vi "Add Frame.vi"(7 "Highlight? (F)":bool, 8 "error in":errorcluster, 10 "Name":string, 11 "Port Ref":T1 format="%.0x") -> (0 "error out":errorcluster, 2 "Newly Created?":bool, 3 "Frame Ref out":T1 format="%.0x")   [LabVIEW 2020, in "Ballard ARINC 429 Scripting.lvlib"]
uses:
  Ballard ARINC 429 Scripting.lvlib
  <vilib>/NI VeriStand/Custom Device API/Custom Device Item Ref.ctl
  Constants.vi
  <vilib>/NI VeriStand/Custom Device API/Custom Device API.lvlib
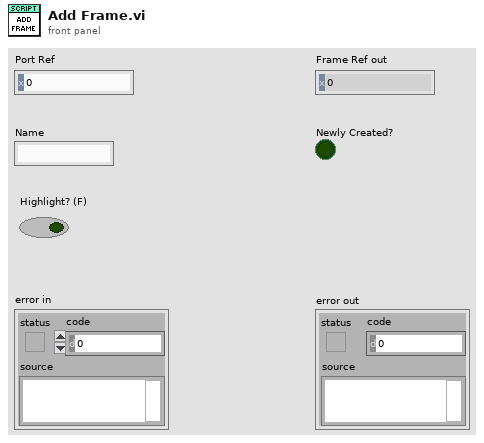
[diagram p1: front panel]
types:
  T1 = typedef "Custom Device API.lvlib/Custom Device Item Ref.ctl" = u64
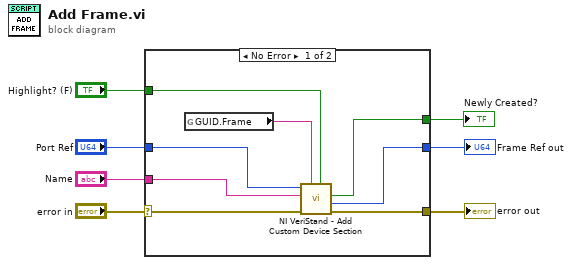
[diagram p0: block diagram]
diagram:
  n1 = case shown="No Error" "error in" {
    selector: "error in" -> [w15 w16]
    tunnel: [w14 w16] -> w6
    tunnel: "Port Ref" -> [w12 _]
    tunnel: [w11 _] -> w4
    tunnel: "Name" -> [w13 _]
    tunnel: "Highlight? (F)" -> [w10 _]
    tunnel: [w9 _] -> w1
    frame No Error {
      n2 = global read "Constants.vi" "GUID.Frame"() -> (w8:string)
      n3 = call <vilib>:"NI VeriStand - Add Custom Device Section.vi"("Highlight? (F)"=w10, "GUID (Default Section)"=w8, "error in (no error)"=w15, "Section Name"=w13, "Parent Ref in"=w12) -> ("error out"=w14:errorcluster, "Section Ptr"=w11:T1, "Newly Created?"=w9:bool)  [unwired: 3 in, 1 out]
    }
    frame Error {
    }
  }
  "Frame Ref out" <- w4
  "error out" <- w6
  "Newly Created?" <- w1
